vi "99.vi"() -> ()   [LabVIEW 2021]
panel:
  out "Array 2":i32[](array[numeric])
  out "Array":T1(array[cluster])
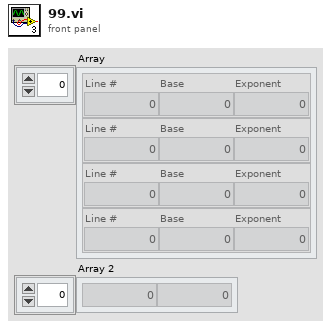
[diagram p1: front panel]
types:
  T1 = cluster{"Line #":i32, "Base":u64, "Exponent":u64}[]
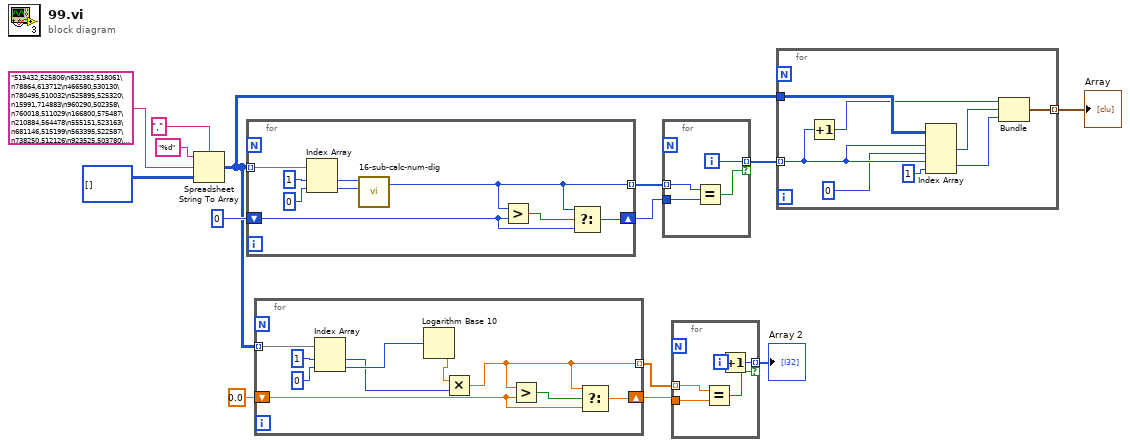
[diagram p0: block diagram]
diagram:
  n1 = Spreadsheet String To Array(delimiter (Tab)=",", format string="%d", spreadsheet string="519432,525806\n632382,518061\n78864,613712\n466580,530130\n780495,510032\n525895,525320\n15991,714883\n960290,502358\n760018,511029\n166800,575487\n210884,564478\n555151,523163\n681146,515199\n563395,522587\n738250,512126\n923525,503780\n595148,520429\n177108,572629\n750923,511482\n440902,532446\n881418,505504\n422489,534197\n979858,501616\n685893,514935\n747477,511661\n167214,575367\n234140,559696\n940238,503122\n728969,512609\n232083,560102\n900971,504694\n688801,514772\n189664,569402\n891022,505104\n445689,531996\n119570,591871\n821453,508118\n371084,539600\n911745,504251\n623655,518600\n144361,582486\n352442,541775\n420726,534367\n295298,549387\n6530,787777\n468397,529976\n672336,515696\n431861,533289\n84228,610150\n805376,508857\n444409,532117\n33833,663511\n381850,538396\n402931,536157\n92901,604930\n304825,548004\n731917,512452\n753734,511344\n51894,637373\n151578,580103\n295075,549421\n303590,548183\n333594,544123\n683952,515042\n60090,628880\n951420,502692\n28335,674991\n714940,513349\n343858,542826\n549279,523586\n804571,508887\n260653,554881\n291399,549966\n402342,536213\n408889,535550\n40328,652524\n375856,539061\n768907,510590\n165993,575715\n976327,501755\n898500,504795\n360404,540830\n478714,529095\n694144,514472\n488726,528258\n841380,507226\n328012,544839\n22389,690868\n604053,519852\n329514,544641\n772965,510390\n492798,527927\n30125,670983\n895603,504906\n450785,531539\n840237,507276\n380711,538522\n63577,625673\n76801,615157\n502694,527123\n597706,520257\n310484,547206\n944468,502959\n121283,591152\n451131,531507\n566499,522367\n425373,533918\n40240,652665\n39130,654392\n714926,513355\n469219,529903\n806929,508783\n287970,550487\n92189,605332\n103841,599094\n671839,515725\n452048,531421\n987837,501323\n935192,503321\n88585,607450\n613883,519216\n144551,582413\n647359,517155\n213902,563816\n184120,570789\n258126,555322\n502546,527130\n407655,535678\n401528,536306\n477490,529193\n841085,507237\n732831,512408\n833000,507595\n904694,504542\n581435,521348\n455545,531110\n873558,505829\n94916,603796\n720176,513068\n545034,523891\n246348,557409\n556452,523079\n832015,507634\n173663,573564\n502634,527125\n250732,556611\n569786,522139\n216919,563178\n521815,525623\n92304,605270\n164446,576167\n753413,511364\n11410,740712\n448845,531712\n925072,503725\n564888,522477\n7062,780812\n641155,517535\n738878,512100\n636204,517828\n372540,539436\n443162,532237\n571192,522042\n655350,516680\n299741,548735\n581914,521307\n965471,502156\n513441,526277\n808682,508700\n237589,559034\n543300,524025\n804712,508889\n247511,557192\n543486,524008\n504383,526992\n326529,545039\n792493,509458\n86033,609017\n126554,589005\n579379,521481\n948026,502823\n404777,535969\n265767,554022\n266876,553840\n46631,643714\n492397,527958\n856106,506581\n795757,509305\n748946,511584\n294694,549480\n409781,535463\n775887,510253\n543747,523991\n210592,564536\n517119,525990\n520253,525751\n247926,557124\n592141,520626\n346580,542492\n544969,523902\n506501,526817\n244520,557738\n144745,582349\n69274,620858\n292620,549784\n926027,503687\n736320,512225\n515528,526113\n407549,535688\n848089,506927\n24141,685711\n9224,757964\n980684,501586\n175259,573121\n489160,528216\n878970,505604\n969546,502002\n525207,525365\n690461,514675\n156510,578551\n659778,516426\n468739,529945\n765252,510770\n76703,615230\n165151,575959\n29779,671736\n928865,503569\n577538,521605\n927555,503618\n185377,570477\n974756,501809\n800130,509093\n217016,563153\n365709,540216\n774508,510320\n588716,520851\n631673,518104\n954076,502590\n777828,510161\n990659,501222\n597799,520254\n786905,509727\n512547,526348\n756449,511212\n869787,505988\n653747,516779\n84623,609900\n839698,507295\n30159,670909\n797275,509234\n678136,515373\n897144,504851\n989554,501263\n413292,535106\n55297,633667\n788650,509637\n486748,528417\n150724,580377\n56434,632490\n77207,614869\n588631,520859\n611619,519367\n100006,601055\n528924,525093\n190225,569257\n851155,506789\n682593,515114\n613043,519275\n514673,526183\n877634,505655\n878905,505602\n1926,914951\n613245,519259\n152481,579816\n841774,507203\n71060,619442\n865335,506175\n90244,606469\n302156,548388\n399059,536557\n478465,529113\n558601,522925\n69132,620966\n267663,553700\n988276,501310\n378354,538787\n529909,525014\n161733,576968\n758541,511109\n823425,508024\n149821,580667\n269258,553438\n481152,528891\n120871,591322\n972322,501901\n981350,501567\n676129,515483\n950860,502717\n119000,592114\n392252,537272\n191618,568919\n946699,502874\n289555,550247\n799322,509139\n703886,513942\n194812,568143\n261823,554685\n203052,566221\n217330,563093\n734748,512313\n391759,537328\n807052,508777\n564467,522510\n59186,629748\n113447,594545\n518063,525916\n905944,504492\n613922,519213\n439093,532607\n445946,531981\n230530,560399\n297887,549007\n459029,530797\n403692,536075\n855118,506616\n963127,502245\n841711,507208\n407411,535699\n924729,503735\n914823,504132\n333725,544101\n176345,572832\n912507,504225\n411273,535308\n259774,555036\n632853,518038\n119723,591801\n163902,576321\n22691,689944\n402427,536212\n175769,572988\n837260,507402\n603432,519893\n313679,546767\n538165,524394\n549026,523608\n61083,627945\n898345,504798\n992556,501153\n369999,539727\n32847,665404\n891292,505088\n152715,579732\n824104,507997\n234057,559711\n730507,512532\n960529,502340\n388395,537687\n958170,502437\n57105,631806\n186025,570311\n993043,501133\n576770,521664\n215319,563513\n927342,503628\n521353,525666\n39563,653705\n752516,511408\n110755,595770\n309749,547305\n374379,539224\n919184,503952\n990652,501226\n647780,517135\n187177,570017\n168938,574877\n649558,517023\n278126,552016\n162039,576868\n658512,516499\n498115,527486\n896583,504868\n561170,522740\n747772,511647\n775093,510294\n652081,516882\n724905,512824\n499707,527365\n47388,642755\n646668,517204\n571700,522007\n180430,571747\n710015,513617\n435522,532941\n98137,602041\n759176,511070\n486124,528467\n526942,525236\n878921,505604\n408313,535602\n926980,503640\n882353,505459\n566887,522345\n3326,853312\n911981,504248\n416309,534800\n392991,537199\n622829,518651\n148647,581055\n496483,527624\n666314,516044\n48562,641293\n672618,515684\n443676,532187\n274065,552661\n265386,554079\n347668,542358\n31816,667448\n181575,571446\n961289,502320\n365689,540214\n987950,501317\n932299,503440\n27388,677243\n746701,511701\n492258,527969\n147823,581323\n57918,630985\n838849,507333\n678038,515375\n27852,676130\n850241,506828\n818403,508253\n131717,587014\n850216,506834\n904848,504529\n189758,569380\n392845,537217\n470876,529761\n925353,503711\n285431,550877\n454098,531234\n823910,508003\n318493,546112\n766067,510730\n261277,554775\n421530,534289\n694130,514478\n120439,591498\n213308,563949\n854063,506662\n365255,540263\n165437,575872\n662240,516281\n289970,550181\n847977,506933\n546083,523816\n413252,535113\n975829,501767\n361540,540701\n235522,559435\n224643,561577\n736350,512229\n328303,544808\n35022,661330\n307838,547578\n474366,529458\n873755,505819\n73978,617220\n827387,507845\n670830,515791\n326511,545034\n309909,547285\n400970,536363\n884827,505352\n718307,513175\n28462,674699\n599384,520150\n253565,556111\n284009,551093\n343403,542876\n446557,531921\n992372,501160\n961601,502308\n696629,514342\n919537,503945\n894709,504944\n892201,505051\n358160,541097\n448503,531745\n832156,507636\n920045,503924\n926137,503675\n416754,534757\n254422,555966\n92498,605151\n826833,507873\n660716,516371\n689335,514746\n160045,577467\n814642,508425\n969939,501993\n242856,558047\n76302,615517\n472083,529653\n587101,520964\n99066,601543\n498005,527503\n709800,513624\n708000,513716\n20171,698134\n285020,550936\n266564,553891\n981563,501557\n846502,506991\n334,1190800\n209268,564829\n9844,752610\n996519,501007\n410059,535426\n432931,533188\n848012,506929\n966803,502110\n983434,501486\n160700,577267\n504374,526989\n832061,507640\n392825,537214\n443842,532165\n440352,532492\n745125,511776\n13718,726392\n661753,516312\n70500,619875\n436952,532814\n424724,533973\n21954,692224\n262490,554567\n716622,513264\n907584,504425\n60086,628882\n837123,507412\n971345,501940\n947162,502855\n139920,584021\n68330,621624\n666452,516038\n731446,512481\n953350,502619\n183157,571042\n845400,507045\n651548,516910\n20399,697344\n861779,506331\n629771,518229\n801706,509026\n189207,569512\n737501,512168\n719272,513115\n479285,529045\n136046,585401\n896746,504860\n891735,505067\n684771,514999\n865309,506184\n379066,538702\n503117,527090\n621780,518717\n209518,564775\n677135,515423\n987500,501340\n197049,567613\n329315,544673\n236756,559196\n357092,541226\n520440,525733\n213471,563911\n956852,502490\n702223,514032\n404943,535955\n178880,572152\n689477,514734\n691351,514630\n866669,506128\n370561,539656\n739805,512051\n71060,619441\n624861,518534\n261660,554714\n366137,540160\n166054,575698\n601878,519990\n153445,579501\n279899,551729\n379166,538691\n423209,534125\n675310,515526\n145641,582050\n691353,514627\n917468,504026\n284778,550976\n81040,612235\n161699,576978\n616394,519057\n767490,510661\n156896,578431\n427408,533714\n254849,555884\n737217,512182\n897133,504851\n203815,566051\n270822,553189\n135854,585475\n778805,510111\n784373,509847\n305426,547921\n733418,512375\n732087,512448\n540668,524215\n702898,513996\n628057,518328\n640280,517587\n422405,534204\n10604,746569\n746038,511733\n839808,507293\n457417,530938\n479030,529064\n341758,543090\n620223,518824\n251661,556451\n561790,522696\n497733,527521\n724201,512863\n489217,528217\n415623,534867\n624610,518548\n847541,506953\n432295,533249\n400391,536421\n961158,502319\n139173,584284\n421225,534315\n579083,521501\n74274,617000\n701142,514087\n374465,539219\n217814,562985\n358972,540995\n88629,607424\n288597,550389\n285819,550812\n538400,524385\n809930,508645\n738326,512126\n955461,502535\n163829,576343\n826475,507891\n376488,538987\n102234,599905\n114650,594002\n52815,636341\n434037,533082\n804744,508880\n98385,601905\n856620,506559\n220057,562517\n844734,507078\n150677,580387\n558697,522917\n621751,518719\n207067,565321\n135297,585677\n932968,503404\n604456,519822\n579728,521462\n244138,557813\n706487,513800\n711627,513523\n853833,506674\n497220,527562\n59428,629511\n564845,522486\n623621,518603\n242689,558077\n125091,589591\n363819,540432\n686453,514901\n656813,516594\n489901,528155\n386380,537905\n542819,524052\n243987,557841\n693412,514514\n488484,528271\n896331,504881\n336730,543721\n728298,512647\n604215,519840\n153729,579413\n595687,520398\n540360,524240\n245779,557511\n924873,503730\n509628,526577\n528523,525122\n3509,847707\n522756,525555\n895447,504922\n44840,646067\n45860,644715\n463487,530404\n398164,536654\n894483,504959\n619415,518874\n966306,502129\n990922,501212\n835756,507474\n548881,523618\n453578,531282\n474993,529410\n80085,612879\n737091,512193\n50789,638638\n979768,501620\n792018,509483\n665001,516122\n86552,608694\n462772,530469\n589233,520821\n891694,505072\n592605,520594\n209645,564741\n42531,649269\n554376,523226\n803814,508929\n334157,544042\n175836,572970\n868379,506051\n658166,516520\n278203,551995\n966198,502126\n627162,518387\n296774,549165\n311803,547027\n843797,507118\n702304,514032\n563875,522553\n33103,664910\n191932,568841\n543514,524006\n506835,526794\n868368,506052\n847025,506971\n678623,515342\n876139,505726\n571997,521984\n598632,520198\n213590,563892\n625404,518497\n726508,512738\n689426,514738\n332495,544264\n411366,535302\n242546,558110\n315209,546555\n797544,509219\n93889,604371\n858879,506454\n124906,589666\n449072,531693\n235960,559345\n642403,517454\n720567,513047\n705534,513858\n603692,519870\n488137,528302\n157370,578285\n63515,625730\n666326,516041\n619226,518883\n443613,532186\n597717,520257\n96225,603069\n86940,608450\n40725,651929\n460976,530625\n268875,553508\n270671,553214\n363254,540500\n384248,538137\n762889,510892\n377941,538833\n278878,551890\n176615,572755\n860008,506412\n944392,502967\n608395,519571\n225283,561450\n45095,645728\n333798,544090\n625733,518476\n995584,501037\n506135,526853\n238050,558952\n557943,522972\n530978,524938\n634244,517949\n177168,572616\n85200,609541\n953043,502630\n523661,525484\n999295,500902\n840803,507246\n961490,502312\n471747,529685\n380705,538523\n911180,504275\n334149,544046\n478992,529065\n325789,545133\n335884,543826\n426976,533760\n749007,511582\n667067,516000\n607586,519623\n674054,515599\n188534,569675\n565185,522464\n172090,573988\n87592,608052\n907432,504424\n8912,760841\n928318,503590\n757917,511138\n718693,513153\n315141,546566\n728326,512645\n353492,541647\n638429,517695\n628892,518280\n877286,505672\n620895,518778\n385878,537959\n423311,534113\n633501,517997\n884833,505360\n883402,505416\n999665,500894\n708395,513697\n548142,523667\n756491,511205\n987352,501340\n766520,510705\n591775,520647\n833758,507563\n843890,507108\n925551,503698\n74816,616598\n646942,517187\n354923,541481\n256291,555638\n634470,517942\n930904,503494\n134221,586071\n282663,551304\n986070,501394\n123636,590176\n123678,590164\n481717,528841\n423076,534137\n866246,506145\n93313,604697\n783632,509880\n317066,546304\n502977,527103\n141272,583545\n71708,618938\n617748,518975\n581190,521362\n193824,568382\n682368,515131\n352956,541712\n351375,541905\n505362,526909\n905165,504518\n128645,588188\n267143,553787\n158409,577965\n482776,528754\n628896,518282\n485233,528547\n563606,522574\n111001,595655\n115920,593445\n365510,540237\n959724,502374\n938763,503184\n930044,503520\n970959,501956\n913658,504176\n68117,621790\n989729,501253\n567697,522288\n820427,508163\n54236,634794\n291557,549938\n124961,589646\n403177,536130\n405421,535899\n410233,535417\n815111,508403\n213176,563974\n83099,610879\n998588,500934\n513640,526263\n129817,587733\n1820,921851\n287584,550539\n299160,548820\n860621,506386\n529258,525059\n586297,521017\n953406,502616\n441234,532410\n986217,501386\n781938,509957\n461247,530595\n735424,512277\n146623,581722\n839838,507288\n510667,526494\n935085,503327\n737523,512167\n303455,548204\n992779,501145\n60240,628739\n939095,503174\n794368,509370\n501825,527189\n459028,530798\n884641,505363\n512287,526364\n835165,507499\n307723,547590\n160587,577304\n735043,512300\n493289,527887\n110717,595785\n306480,547772\n318593,546089\n179810,571911\n200531,566799\n314999,546580\n197020,567622\n301465,548487\n237808,559000\n131944,586923\n882527,505449\n468117,530003\n711319,513541\n156240,578628\n965452,502162\n992756,501148\n437959,532715\n739938,512046\n614249,519196\n391496,537356\n62746,626418\n688215,514806\n75501,616091\n883573,505412\n558824,522910\n759371,511061\n173913,573489\n891351,505089\n727464,512693\n164833,576051\n812317,508529\n540320,524243\n698061,514257\n69149,620952\n471673,529694\n159092,577753\n428134,533653\n89997,606608\n711061,513557\n779403,510081\n203327,566155\n798176,509187\n667688,515963\n636120,517833\n137410,584913\n217615,563034\n556887,523038\n667229,515991\n672276,515708\n325361,545187\n172115,573985\n13846,725685", array type (2D Dbl)=u64[][] []) -> (array=w5:u64[][])
  n2 = for {
    tunnel: w5 -> [w23] mode=indexing
    shift-right: [w16] -> w8
    shift-left: 0 -> [w17]
    tunnel: [w15] -> w9 mode=indexing
    n3 = Index Array(array=w23, index #1=1 ("index"), index #2=0 ("index")) -> (element #1=w20:u64, element #2=w19:u64)
    n4 = call "16-sub-calc-num-dig.vi"("base in"=w19, "exponent in"=w20) -> ("Number of Digits"=w15:i32)  [unwired: 3 in]
    n5 = Greater?(x=w15, y=w17) -> (0:w18:bool)
    n6 = Select(t=w15, s=w18, f=w17) -> (s? t:f=w16:i32)
  }
  n7 = for {
    tunnel: w5 -> [w33] mode=indexing
    shift-right: [w28] -> w3
    shift-left: 0.0 -> [w29]
    tunnel: [w24] -> w2 mode=indexing
    n8 = Index Array(array=w33, index #1=1 ("index"), index #2=0 ("index")) -> (element #1=w25:u64, element #2=w27:u64)
    n9 = Logarithm Base 10(1:w27) -> (0:w26:dbl)
    n10 = Multiply(x=w26, y=w25) -> (x*y=w24:dbl)
    n11 = Greater?(x=w24, y=w29) -> (0:w30:bool)
    n12 = Select(t=w24, s=w30, f=w29) -> (s? t:f=w28:dbl)
  }
  n13 = for {
    tunnel: [w37] -> w7 mode=indexing if=w34
    tunnel: w9 -> [w36] mode=indexing
    tunnel: w8 -> [w35]
    i -> [w37]
    n14 = Equal?(x=w36, y=w35) -> (x = y?=w34:bool)
  }
  n15 = for {
    tunnel: [w38] -> w1 mode=indexing if=w39
    tunnel: w2 -> [w41] mode=indexing
    tunnel: w3 -> [w40]
    i -> [w42]
    n16 = Equal?(x=w41, y=w40) -> (x = y?=w39:bool)
    n17 = Increment(x=w42) -> (x+1=w38:i32)
  }
  "Array 2" <- w1
  n18 = for {
    tunnel: w5 -> [w50]
    tunnel: w7 -> [w49] mode=indexing
    tunnel: [w43] -> w6 mode=indexing
    n19 = Increment(x=w49) -> (x+1=w48:i32)
    n20 = Index Array(array=w50, index (row) #1=w49, index (col) #1=0 ("disabled index (col)"), index (row) #2=w49, index (col) #2=1 ("disabled index (col)")) -> (element #1=w47:u64, element #2=w44:u64)
    n21 = Bundle(w48, w47, w44) -> (w43:cluster{i32, u64, u64})  [unwired: 1 in]
  }
  "Array" <- w6
